vi "CLSUIP_ShouldReplaceControl.vi"(4 "error in (no error)":errorcluster, 5 "Terminal Index":u32, 6 "ConPane":refnum<vi>, 7 "ElementWrapperRetooler":refnum<class "ElementWrapperRetooler.lvclass">) -> (0 "error out":errorcluster, 1 "Should replace?":bool, 3 "ElementWrapperRetooler out":refnum<class "ElementWrapperRetooler.lvclass">)   [LabVIEW 2021, in "MemberVICreation.lvlib" / "ElementWrapperRetooler.lvclass"]
uses:
  <resource>/Framework/Providers/LVClassLibrary/NewAccessors/ElementWrapperRetooler/ElementWrapperRetooler.lvclass
  c:/dev/_r/3/eng/lv-core/lvpostprocessingd/labview_english/dist_i386/resource/Framework/Providers/LVClassLibrary/NewAccessors/VIRetooler/VIRetooler.lvclass
  <resource>/Framework/Providers/LVClassLibrary/NewAccessors/VIRetooler/VIRetooler.lvclass
  <vilib>/Utility/VariantDataType/VariantType.lvlib
  <resource>/Framework/Providers/LVClassLibrary/NewAccessors/MemberVICreation.lvlib
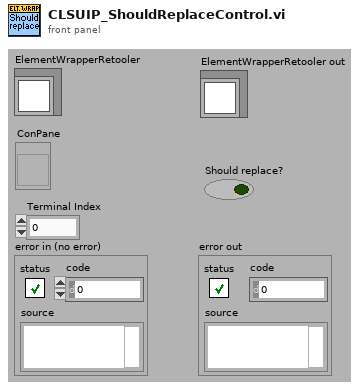
[diagram p1: front panel]
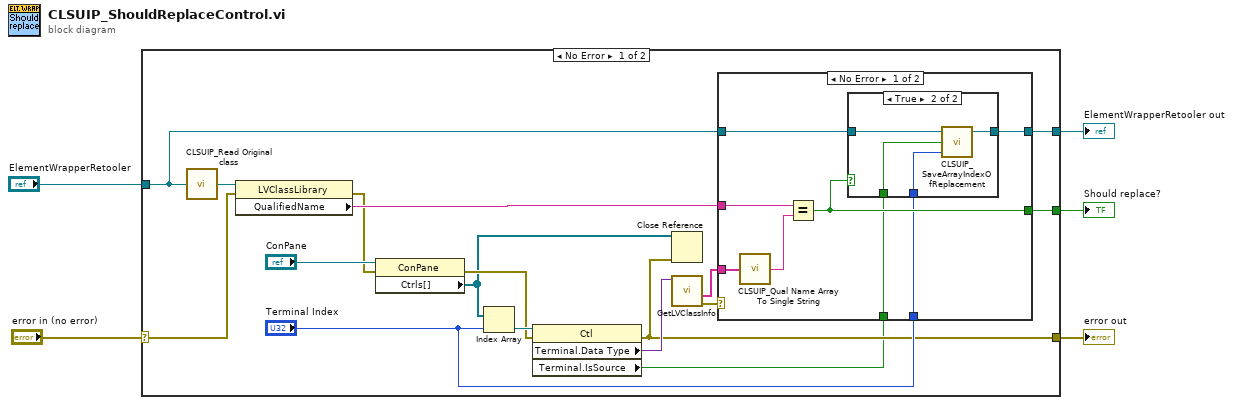
[diagram p0: block diagram]
diagram:
  n1 = case shown="No Error" "error in (no error)" {
    selector: "error in (no error)" -> [w6 w38]
    tunnel: [w8 w38] -> w4
    tunnel: [w18 _] -> w3
    tunnel: "ElementWrapperRetooler" -> [w12 w37]
    tunnel: [w11 w37] -> w1
    frame No Error {
      n2 = call <resource>:"CLSUIP_Read Original class.vi"("VIRetooler.lvclass in"=w12) -> ("Orig class"=w15:refnum<vi>)
      n3 = property class="LVClassLibrary"(reference=w15, error in=w6) -> (error out=w13:errorcluster, "QualifiedName"=w14:string)  [unwired: 1 out]
      n4 = property class="ConPane"(reference="ConPane", error in=w13) -> (error out=w17:errorcluster, "Ctrls[]"=w9:refnum<vi>[])  [unwired: 1 out]
      n5 = Index Array(array=w9, index="Terminal Index") -> (element=w21:refnum<vi>)
      n6 = property class="Ctl"(reference=w21, error in=w17) -> (error out=w8:errorcluster, "Terminal.Data Type"=w20:variant, "Terminal.IsSource"=w7:bool)  [unwired: 1 out]
      n7 = Close Reference(reference=w9, error in (no error)=w8) -> ()  [unwired: 1 out]
      n8 = call <vilib>:"GetLVClassInfo.vi"("Variant"=w20) -> ("error out"=w16:errorcluster, "Fully Qualified LV Class Name"=w19:string[])  [unwired: 1 in, 8 out]
      n9 = case shown="No Error" w16 {
        tunnel: w19 -> [w30 _]
        tunnel: [w27 _] -> w18
        tunnel: w14 -> [w28 _]
        tunnel: w12 -> [w26 w36]
        tunnel: "Terminal Index" -> [w25 _]
        tunnel: [w24 w36] -> w11
        tunnel: w7 -> [w23 _]
        frame No Error {
          n10 = call <resource>:"CLSUIP_Qual Name Array To Single String.vi"("Fully Qualified Array"=w30) -> ("Fully Qualified String"=w29:string)
          n11 = Equal?(x=w28, y=w29) -> (x = y?=w27:bool)
          n12 = case shown="True" w27 {
            tunnel: w26 -> [w31 w34]
            tunnel: w25 -> [_ w35]
            tunnel: [w31 w33] -> w24
            tunnel: w23 -> [_ w32]
            frame False {
            }
            frame True {
              n13 = call <resource>:"CLSUIP_SaveArrayIndexOfReplacement.vi"("Terminal Index"=w35, "Terminal.IsSource"=w32, "ElementWrapperRetooler in"=w34) -> ("ElementWrapperRetooler out"=w33:refnum<class "ElementWrapperRetooler.lvclass">)  [unwired: 2 out]
            }
          }
        }
        frame Error {
          # "Don't propagate this error.\nThis just means the control\nis not an LVClass control."
        }
      }
    }
    frame Error {
    }
  }
  "error out" <- w4
  "Should replace?" <- w3
  "ElementWrapperRetooler out" <- w1
